vi "Lvi Subsystem Set Ctr One Shot Repeat Mode.vi"(7 "Polarity":i32, 8 "error in (no error)":errorcluster, 9 "GateEdge":i32, 10 "Millisecs":dbl, 11 "TaskRef":i32) -> (0 "error out":errorcluster, 1 "function return":i32, 2 "ActualMillisecs":dbl, 3 "TaskRef out":i32)   [LabVIEW 2016, in "DtLvLink.lvlib"]
doc: "Calls directly into the entry points of the DLL of the Data Acq SDK to create one or more virtual channels, add them to a task, and configure the task with the specified settings to output a single pulse for a specified duration (in milliseconds) each time that the device detects a trigger (determined by the counter/timer's gate input signal). This VI is used by the higher-level VI, DtOLCreateTask."
uses:
  <userlib>/LV-Link3/DtLvLink.lvlib
  <userlib>/LV-Link3/DtLvLink_32.dll
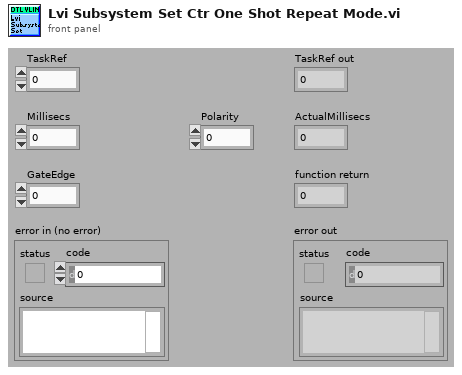
[diagram p1: front panel]
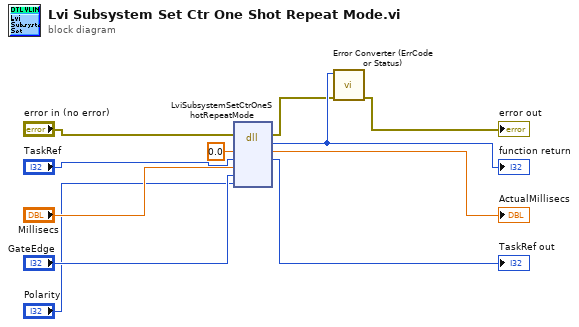
[diagram p0: block diagram]
diagram:
  n1 = dll-call lib="C:/Program Files (x86)/National Instruments/LabVIEW 2016/user.lib/LV-Link3/DtLvLink_32.*" fn="LviSubsystemSetCtrOneShotRepeatMode"(error in="error in (no error)", "ActualMillisecs"=0.0, "TaskRef"="TaskRef", "Millisecs"="Millisecs", "GateEdge"="GateEdge", "Polarity"="Polarity") -> (error out=w2:errorcluster, w11:i32, "ActualMillisecs"=→"ActualMillisecs":dbl, "TaskRef"=→"TaskRef out":i32)  [unwired: 5 in, 1 out]
  "function return" <- w11
  n2 = call <userlib>:"Error Converter (ErrCode or Status).vi"("error in (no error)"=w2, "error code"=w11) -> ("error out"=→"error out":errorcluster)  [unwired: 9 in]
